vi "__SISbias_Set.vi"(6 "SIS@Mode":u16(ring), 8 "Offset":dbl, 9 "Set_V":dbl, 10 "Bias_LO_equip":T1={"Node address"=19, "CAN Interface"="CAN0", "Cartridge band"=10, "Slave Node in"={"Address"=19, "Serial Number"=[16, 71, 55, 76, 1, 8, 0, -15]}, "ObjHandle out"=159055936, "POL"=1, "sb"=1, "GPIB_SM (SIS S,V)"="24", "GPIB_DMM (SIS I)"="22", "GPIB_SM (MAG I) "="25", "GPIB_SG(LO)"="19", "GPIB_PW (PAMP) "="6", "GPIB_TMP1(8ch)"="12", "GPIB_TMP2(2ch)  "="13", "WCA_avg"=10, "Rsen"=10.0, "BiasModule"=0, "LOModule "=4, "WCA_LO_FREQ_SET"={"YTO Low freq. [GHz]"=14.42, "YTO High freq. [GHz]"=17.7, "Kvco"=1, "Lock Pol."=0, "SET LO FREQ"=72.5, "Multiplier"=6.0, "YTO (HEX)"=0, "YTO coarse( FREQ)"=25.0, "NULL PLL INTEGRATOR"=FALSE}, "Res for"=0} {"Res for" items=["none", "series res", "parallel res"]; "WCA_LO_FREQ_SET"."YTO coarse( FREQ)" min=25 max=150 step=0.0001 format="%.3f"; "WCA_LO_FREQ_SET"."Multiplier" min=3 max=6 step=3; "WCA_LO_FREQ_SET"."SET LO FREQ" min=25 max=150 step=0.0001 format="%.3f"; "WCA_LO_FREQ_SET"."Lock Pol." items=["Lower", "Upper"]; "WCA_LO_FREQ_SET"."Kvco" items=["7.5MHz/V", "15MHz/V"]; "WCA_LO_FREQ_SET"."YTO High freq. [GHz]" format="%.3f"; "WCA_LO_FREQ_SET"."YTO Low freq. [GHz]" format="%.3f"; "LOModule" items=["Manual Gunn+PAMP"=0, "B10Lab LO"=1, "WCA LO"=2, ""=3, "YIGtransmitter"=4, "none"=99]; "BiasModule" items=["B10Lab Bias"=0, "WCA BiasModule"=1, "none"=99]; "Slave Node in"."Serial Number" format="%.0x"; "Slave Node in"."Address" format="%.0x"; "Cartridge band" max=10 step=1; "Node address" format="%.0x"}) -> (0 "error out":errorcluster caption="Error out")   [LabVIEW 2017]
panel:
  # "LO freq. [GHz]"
  # "YTO LOW\n/High Freq."
  # "ZERO Intgrtr"
  # "Node Address"
  # "Serial Number"
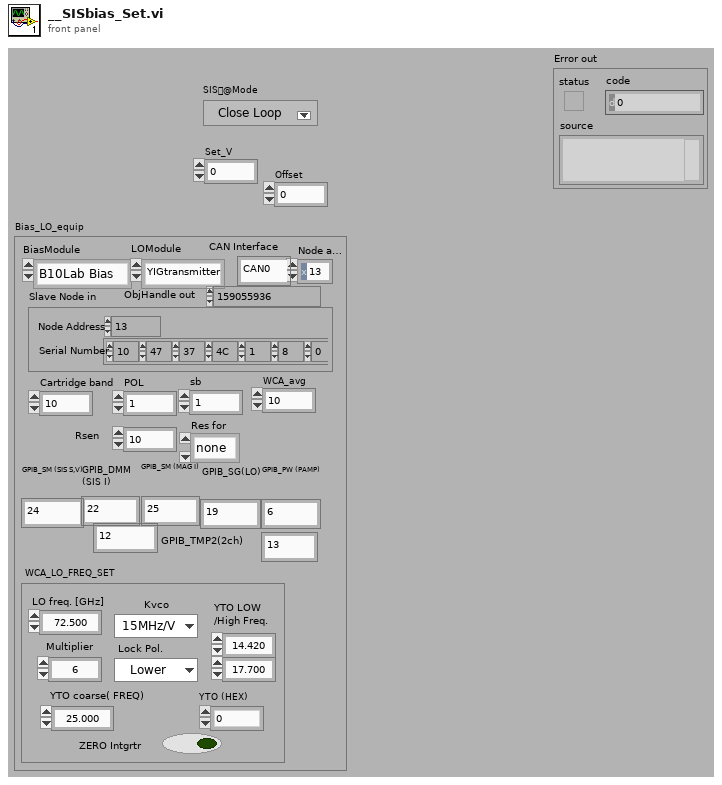
[diagram p1: front panel]
types:
  T1 = cluster{"Node address":u16, "CAN Interface":string, "Cartridge band":u32, "Slave Node in":cluster{"Address":i16, "Serial Number":i8[]}, "ObjHandle out":u32, "POL":u32, "sb":u32, "GPIB_SM (SIS S,V)":string, "GPIB_DMM (SIS I)":string, "GPIB_SM (MAG I) ":string, "GPIB_SG(LO)":string, "GPIB_PW (PAMP) ":string, "GPIB_TMP1(8ch)":string, "GPIB_TMP2(2ch)  ":string, "WCA_avg":i32, "Rsen":dbl, "BiasModule":u16, "LOModule ":u16, "WCA_LO_FREQ_SET":cluster{"YTO Low freq. [GHz]":sgl, "YTO High freq. [GHz]":sgl, "Kvco":u16, "Lock Pol.":u16, "SET LO FREQ":sgl, "Multiplier":sgl, "YTO (HEX)":u16, "YTO coarse( FREQ)":sgl, "NULL PLL INTEGRATOR":bool}, "Res for":u16}
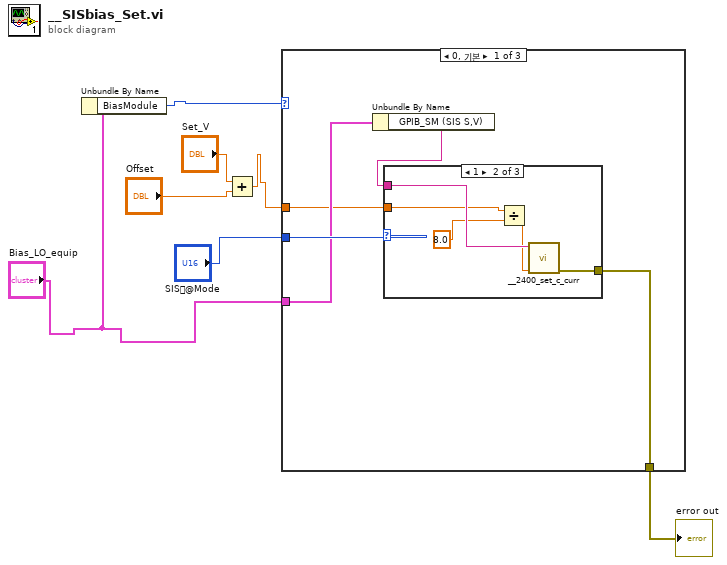
[diagram p0: block diagram]
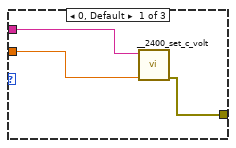
[diagram p2: hidden frame]
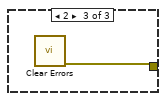
[diagram p3: hidden frame]
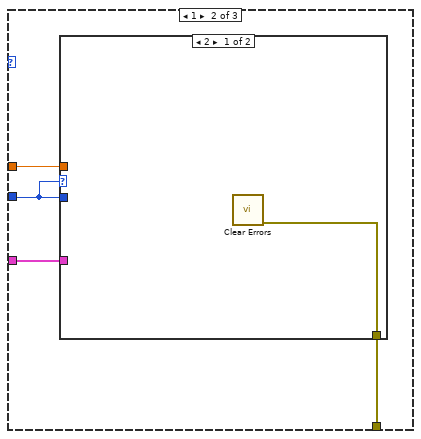
[diagram p4: hidden frame]
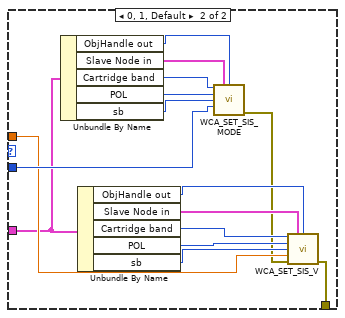
[diagram p5: hidden frame]
diagram:
  n1 = Unbundle By Name("Bias_LO_equip") -> ("BiasModule"=w2:u16)
  n2 = Add(x="Set_V", y="Offset") -> (x+y=w4:dbl)
  n3 = case shown="0, 기본" w2 {
    tunnel: "SIS@Mode" -> [w12 w22 _]
    tunnel: "Bias_LO_equip" -> [w11 w24 _]
    tunnel: w4 -> [w10 w25 _]
    tunnel: [w8 w23 _] -> w3
    frame 0, Default {
      n4 = Unbundle By Name(w11) -> ("GPIB_SM (SIS S,V)"=w9:string)
      n5 = case shown="1" w12 {
        tunnel: w9 -> [w15 w20 _]
        tunnel: w10 -> [w14 w18 _]
        tunnel: [w13 w16 w21] -> w8
        frame 0, Default {
          n6 = call "__2400_set_c_volt.vi"("volt_set(mV)"=w14, "GPIB"=w15) -> ("error out"=w13:errorcluster)  [unwired: 5 in]
        }
        frame 1 {
          n7 = Divide(x=w18, y=8.0) -> (x/y=w19:dbl)
          n8 = call "__2400_set_c_curr.vi"("curr_set(mA)"=w19, "GPIB"=w20) -> ("error out"=w16:errorcluster)  [unwired: 5 in]
        }
        frame 2 {
          n9 = call <vilib>:"Clear Errors.vi"() -> ("error out"=w21:errorcluster)  [unwired: 6 in, 1 out]
        }
      }
    }
    frame 1 {
      n10 = case shown="2" w22 {
        tunnel: w22 -> [_ w36]
        tunnel: w25 -> [_ w30]
        tunnel: w24 -> [_ w28]
        tunnel: [w26 w27] -> w23
        frame 2 {
          n11 = call <vilib>:"Clear Errors.vi"() -> ("error out"=w26:errorcluster)  [unwired: 6 in, 1 out]
        }
        frame 0, 1, Default {
          n12 = Unbundle By Name(w28) -> ("ObjHandle out"=w41:u32, "Slave Node in"=w40:cluster{"Address":i16, "Serial Number":i8[]}, "Cartridge band"=w39:u32, "POL"=w38:u32, "sb"=w37:u32)
          n13 = Unbundle By Name(w28) -> ("ObjHandle out"=w31:u32, "Slave Node in"=w32:cluster{"Address":i16, "Serial Number":i8[]}, "Cartridge band"=w33:u32, "POL"=w34:u32, "sb"=w35:u32)
          n14 = call "WCA_SET_SIS_MODE.vi"("Cartridge Band"=w39, "Slave Node in"=w40, "ObjHandle in"=w41, "POL"=w38, "sb"=w37, "SET_SIS_MODE"=w36) -> ("error out"=w29:errorcluster)  [unwired: 8 in, 1 out]
          n15 = call "WCA_SET_SIS_V.vi"("Cartridge Band"=w33, "Slave Node in"=w32, "ObjHandle in"=w31, "POL"=w34, "sb"=w35, "SET_SIS_V"=w30, "error in (no error)"=w29) -> ("error out"=w27:errorcluster)  [unwired: 7 in, 1 out]
        }
      }
    }
    frame 99 {
    }
  }
  "error out" <- w3
